vi "Backlash (DBL).vi"(1 "reinitialize? (F)":bool, 2 "initial output":dbl format="%.2f", 3 "deadband":dbl=1.0 format="%.2f", 4 "input":dbl format="%.2f") -> (0 "output":dbl format="%.2f")   [LabVIEW 2020, in "NI_AdvCtrl_nonlinear.lvlib"]
doc: "LabVIEW no longer supports this VI. You can obtain similar functionality by installing the LabVIEW Simulation Module.\n\nImplements a backlash or deadband function. Output will not change until the input value differs from the current output by at least the deadband amount."
uses:
  <vilib>/addons/control/advanced/NI_AdvCtrl_nonlinear.lvlib
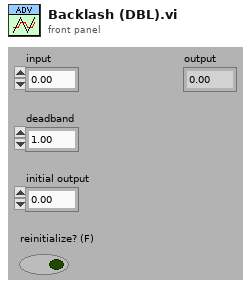
[diagram p1: front panel]
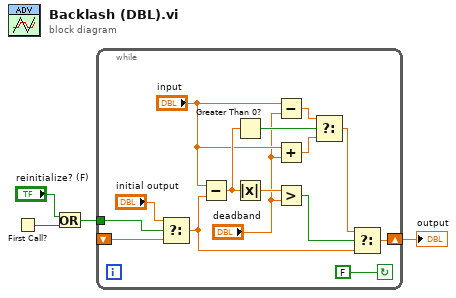
[diagram p0: block diagram]
diagram:
  n1 = First Call?() -> (First Call?: T/F=w3:bool)
  n2 = Or(x="reinitialize? (F)", y=w3) -> (x .or. y?=w1:bool)
  n3 = while {
    tunnel: w1 -> [w5]
    shift-left: _ -> [w6]
    shift-right: [w17] -> w4
    stop <- FALSE continue-if-true
    n4 = Select(t="initial output", s=w5, f=w6) -> (s? t:f=w8:dbl)
    n5 = Subtract(x="input", y=w8) -> (x-y=w16:dbl)
    n6 = Greater Than 0?(x=w16) -> (x > 0?=w15:bool)
    n7 = Absolute Value(x=w16) -> (abs(x)=w19:dbl)
    n8 = Subtract(x="input", y="deadband") -> (x-y=w13:dbl)
    n9 = Add(x="input", y="deadband") -> (x+y=w14:dbl)
    n10 = Greater?(x=w19, y="deadband") -> (0:w18:bool)
    n11 = Select(t=w13, s=w15, f=w14) -> (s? t:f=w12:dbl)
    n12 = Select(t=w12, s=w18, f=w8) -> (s? t:f=w17:dbl)
  }
  "output" <- w4
